vi "AD7609_Reset.vi"   [LabVIEW 2012]
uses:
  <vilib>/rvi/eio/common/nirviEmuTemplateMethod_errors.vi
  <vilib>/eio/EIONode/EIONode.xnode
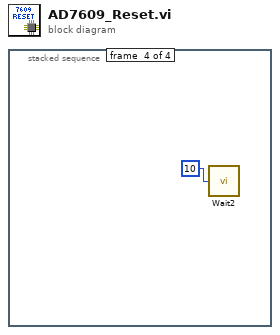
[diagram p0: block diagram]
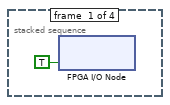
[diagram p2: hidden frame]
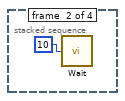
[diagram p3: hidden frame]
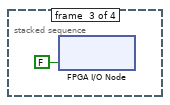
[diagram p4: hidden frame]
diagram:
  n1 = stacked-sequence {
    frame #0 {
      n2 = xnode "FPGA I/O Node"("RESET"=TRUE) -> ()  [unwired: 1 in, 1 out]
    }
    frame #1 {
      n3 = call "Wait"("Count(Ticks)"=u8 10 ("T_reset")) -> ()  [unwired: 1 out]
    }
    frame #2 {
      n4 = xnode "FPGA I/O Node"("RESET"=FALSE) -> ()  [unwired: 1 in, 1 out]
    }
    frame #3 {
      n5 = call "Wait2"("Count(Ticks)"=u8 10 ("D_reset")) -> ()  [unwired: 1 out]
    }
  }
